vi "FPGA_EncoderWriteTimerConfiguration.vi"(8 "error in (no error)":errorcluster, 9 "AverageSize":u8=1, 10 "StallPeriod (sec)":dbl=0.05, 11 "EncoderDevRef":T1) -> (0 "error out":errorcluster, 3 "EncoderDevRef":T1)   [LabVIEW 2017]
uses:
  <vilib>/Rock Robotics/SystemInterfaces/Encoder/FPGA_EncoderDevRef.ctl
  <vilib>/Rock Robotics/SystemInterfaces/Encoder/FPGA_EncoderIdx.ctl
  <vilib>/Rock Robotics/SystemInterfaces/System/FPGA_SystemFPGA Ref Global.vi
  <vilib>/Utility/error.llb/Error Cluster From Error Code.vi
  <vilib>/rvi/errors/niLvFpgaAdjustHostInterfaceError.vi
  <vilib>/rvi/interface/nirviReadWriteControl/nirviReadWriteControl.xnode
  <vilib>/Rock Robotics/SystemInterfaces/System/FPGA_SystemFRC FPGA Ref.ctl
  NiFpgaLv.dll
  <vilib>/rvi/interface/Simulation/niFpgaSimulationCallBeginRW.vi
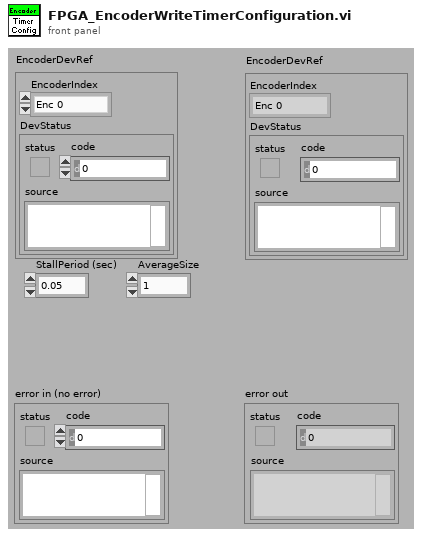
[diagram p1: front panel]
types:
  T1 = typedef "FPGA_EncoderDevRef.ctl" = cluster{"EncoderIndex":T2, "DevStatus":errorcluster}
  T2 = typedef "FPGA_EncoderIdx.ctl" = enum8{"Enc 0", "Enc 1", "Enc 2", "Enc 3", "Enc 4", "Enc 5", "Enc 6", "Enc 7", "Invalid"}
  T3 = typedef "FPGA_SystemFRC FPGA Ref.ctl" = refnum<k20>
  T4 = cluster{"StallPeriod":fxp<+,24,25>, "AverageSize":fxp<+,7,7>, "UpdateWhenEmpty":bool}
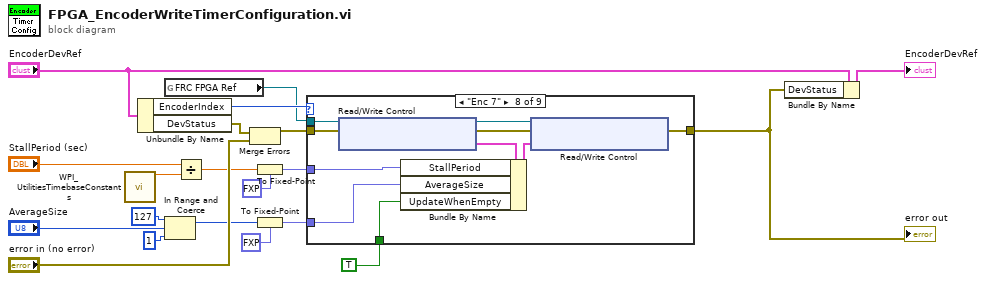
[diagram p0: block diagram]
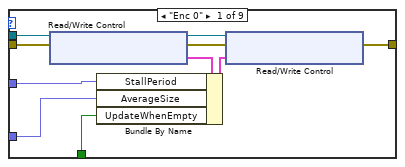
[diagram p2: hidden frame]
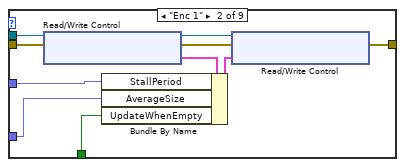
[diagram p3: hidden frame]
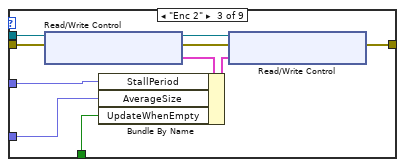
[diagram p4: hidden frame]
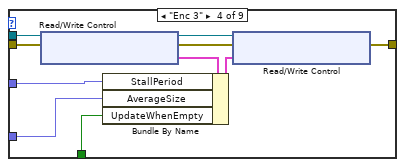
[diagram p5: hidden frame]
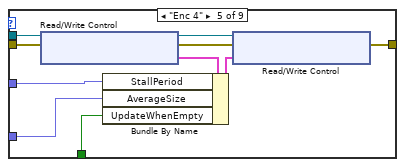
[diagram p6: hidden frame]
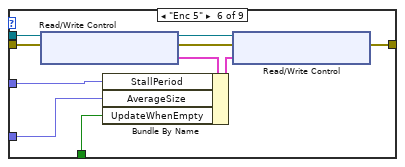
[diagram p7: hidden frame]
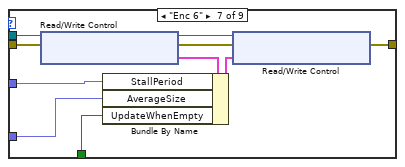
[diagram p8: hidden frame]
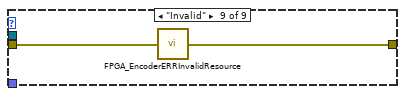
[diagram p9: hidden frame]
diagram:
  n1 = call <vilib>:"WPI_UtilitiesTimebaseConstants.vi"() -> ("40 MHz FPGA clock"=w1:dbl)  [unwired: 13 in, 2 out]
  n2 = Unbundle By Name("EncoderDevRef") -> ("EncoderIndex"=w15:T2, "DevStatus"=w3:errorcluster)
  n3 = global read "FPGA_SystemFPGA Ref Global.vi" "FRC FPGA Ref"() -> (w5:T3)
  n4 = In Range and Coerce(upper limit=u8 127, x="AverageSize", lower limit=u8 1) -> (coerced(x)=w7:u8)  [unwired: 1 out]
  n5 = Divide(x="StallPeriod (sec)", y=w1) -> (x/y=w6:dbl)
  n6 = Merge Errors(w3, "error in (no error)") -> (w4:errorcluster)
  n7 = To Fixed-Point(fixed-point type=fxp<+,24,25> 0.0 ("StallPeriod"), number=w6) -> (fixed-point=w14:fxp<+,24,25>)
  n8 = To Fixed-Point(fixed-point type=fxp<+,7,7> 0.0 ("AverageSize"), number=w7) -> (fixed-point=w11:fxp<+,7,7>)
  n9 = case shown="\"Enc 7\"" w15 {
    tunnel: w5 -> [w27 w38 w47 w58 w68 w78 w88 w98 _]
    tunnel: w4 -> [w26 w37 w48 w57 w67 w77 w87 w97 w102]
    tunnel: [w25 w36 w46 w56 w66 w76 w86 w96 w101] -> w18
    tunnel: w14 -> [w23 w35 w45 w55 w65 w75 w85 w95 _]
    tunnel: w11 -> [w22 w31 w41 w51 w61 w71 w81 w91 _]
    tunnel: TRUE ("UpdateWhenEmpty") -> [w21 w32 w42 w52 w62 w72 w82 w92 _]
    frame "Enc 0" {
      n10 = xnode "Read/Write Control"("FPGA VI Reference In"=w27, "error in"=w26) -> ("FPGA VI Reference Out"=w30:T3, "error out"=w29:errorcluster, "Encoder0.TimerConfig"=w24:T4)
      n11 = Bundle By Name(cluster=w24, "StallPeriod"=w23, "AverageSize"=w22, "UpdateWhenEmpty"=w21) -> (w28:T4)
      n12 = xnode "Read/Write Control"("FPGA VI Reference In"=w30, "error in"=w29, "Encoder0.TimerConfig"=w28) -> ("error out"=w25:errorcluster)  [unwired: 1 out]
    }
    frame "Enc 1" {
      n13 = xnode "Read/Write Control"("FPGA VI Reference In"=w38, "error in"=w37) -> ("FPGA VI Reference Out"=w40:T3, "error out"=w39:errorcluster, "Encoder1.TimerConfig"=w34:T4)
      n14 = Bundle By Name(cluster=w34, "StallPeriod"=w35, "AverageSize"=w31, "UpdateWhenEmpty"=w32) -> (w33:T4)
      n15 = xnode "Read/Write Control"("FPGA VI Reference In"=w40, "error in"=w39, "Encoder1.TimerConfig"=w33) -> ("error out"=w36:errorcluster)  [unwired: 1 out]
    }
    frame "Enc 2" {
      n16 = xnode "Read/Write Control"("FPGA VI Reference In"=w47, "error in"=w48) -> ("FPGA VI Reference Out"=w50:T3, "error out"=w49:errorcluster, "Encoder2.TimerConfig"=w44:T4)
      n17 = Bundle By Name(cluster=w44, "StallPeriod"=w45, "AverageSize"=w41, "UpdateWhenEmpty"=w42) -> (w43:T4)
      n18 = xnode "Read/Write Control"("FPGA VI Reference In"=w50, "error in"=w49, "Encoder2.TimerConfig"=w43) -> ("error out"=w46:errorcluster)  [unwired: 1 out]
    }
    frame "Enc 3" {
      n19 = xnode "Read/Write Control"("FPGA VI Reference In"=w58, "error in"=w57) -> ("FPGA VI Reference Out"=w60:T3, "error out"=w59:errorcluster, "Encoder3.TimerConfig"=w54:T4)
      n20 = Bundle By Name(cluster=w54, "StallPeriod"=w55, "AverageSize"=w51, "UpdateWhenEmpty"=w52) -> (w53:T4)
      n21 = xnode "Read/Write Control"("FPGA VI Reference In"=w60, "error in"=w59, "Encoder3.TimerConfig"=w53) -> ("error out"=w56:errorcluster)  [unwired: 1 out]
    }
    frame "Enc 4" {
      n22 = xnode "Read/Write Control"("FPGA VI Reference In"=w68, "error in"=w67) -> ("FPGA VI Reference Out"=w70:T3, "error out"=w69:errorcluster, "Encoder4.TimerConfig"=w64:T4)
      n23 = Bundle By Name(cluster=w64, "StallPeriod"=w65, "AverageSize"=w61, "UpdateWhenEmpty"=w62) -> (w63:T4)
      n24 = xnode "Read/Write Control"("FPGA VI Reference In"=w70, "error in"=w69, "Encoder4.TimerConfig"=w63) -> ("error out"=w66:errorcluster)  [unwired: 1 out]
    }
    frame "Enc 5" {
      n25 = xnode "Read/Write Control"("FPGA VI Reference In"=w78, "error in"=w77) -> ("FPGA VI Reference Out"=w80:T3, "error out"=w79:errorcluster, "Encoder5.TimerConfig"=w74:T4)
      n26 = Bundle By Name(cluster=w74, "StallPeriod"=w75, "AverageSize"=w71, "UpdateWhenEmpty"=w72) -> (w73:T4)
      n27 = xnode "Read/Write Control"("FPGA VI Reference In"=w80, "error in"=w79, "Encoder5.TimerConfig"=w73) -> ("error out"=w76:errorcluster)  [unwired: 1 out]
    }
    frame "Enc 6" {
      n28 = xnode "Read/Write Control"("FPGA VI Reference In"=w88, "error in"=w87) -> ("FPGA VI Reference Out"=w90:T3, "error out"=w89:errorcluster, "Encoder6.TimerConfig"=w84:T4)
      n29 = Bundle By Name(cluster=w84, "StallPeriod"=w85, "AverageSize"=w81, "UpdateWhenEmpty"=w82) -> (w83:T4)
      n30 = xnode "Read/Write Control"("FPGA VI Reference In"=w90, "error in"=w89, "Encoder6.TimerConfig"=w83) -> ("error out"=w86:errorcluster)  [unwired: 1 out]
    }
    frame "Enc 7" {
      n31 = xnode "Read/Write Control"("FPGA VI Reference In"=w98, "error in"=w97) -> ("FPGA VI Reference Out"=w100:T3, "error out"=w99:errorcluster, "Encoder7.TimerConfig"=w94:T4)
      n32 = Bundle By Name(cluster=w94, "StallPeriod"=w95, "AverageSize"=w91, "UpdateWhenEmpty"=w92) -> (w93:T4)
      n33 = xnode "Read/Write Control"("FPGA VI Reference In"=w100, "error in"=w99, "Encoder7.TimerConfig"=w93) -> ("error out"=w96:errorcluster)  [unwired: 1 out]
    }
    frame "Invalid" {
      n34 = call <vilib>:"FPGA_EncoderERRInvalidResource.vi"("error in (no error)"=w102) -> ("error out"=w101:errorcluster)
    }
  }
  "error out" <- w18
  n35 = Bundle By Name(cluster="EncoderDevRef", "DevStatus"=w18) -> (→"EncoderDevRef":T1)
